vi "final.vi"() -> ()   [LabVIEW 2018]
panel:
  out "RAW\nVOLTAGE":dbl format="%#_3g"
  out "SCALED VOLTAGE":dbl(knob) scale=0.0..10.0
  in  "stop":bool
  out "STATUS":string
  out "ABOVE\nROOM\nTEMP":bool
  out "Numeric":dbl format="%#_3g"
  out "Thermometer":dbl(slide) scale=0.0..400.0
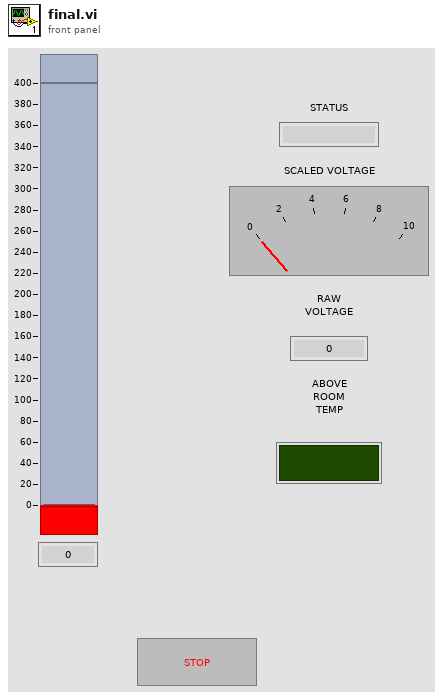
[diagram p1: front panel]
types:
  T1 = cluster{"data[0]":bool, "data[1]":bool, "data[2]":bool, "data[3]":bool, "data[4]":bool, "data[5]":bool, "data[6]":bool, "data[7]":bool, "data[8]":bool}
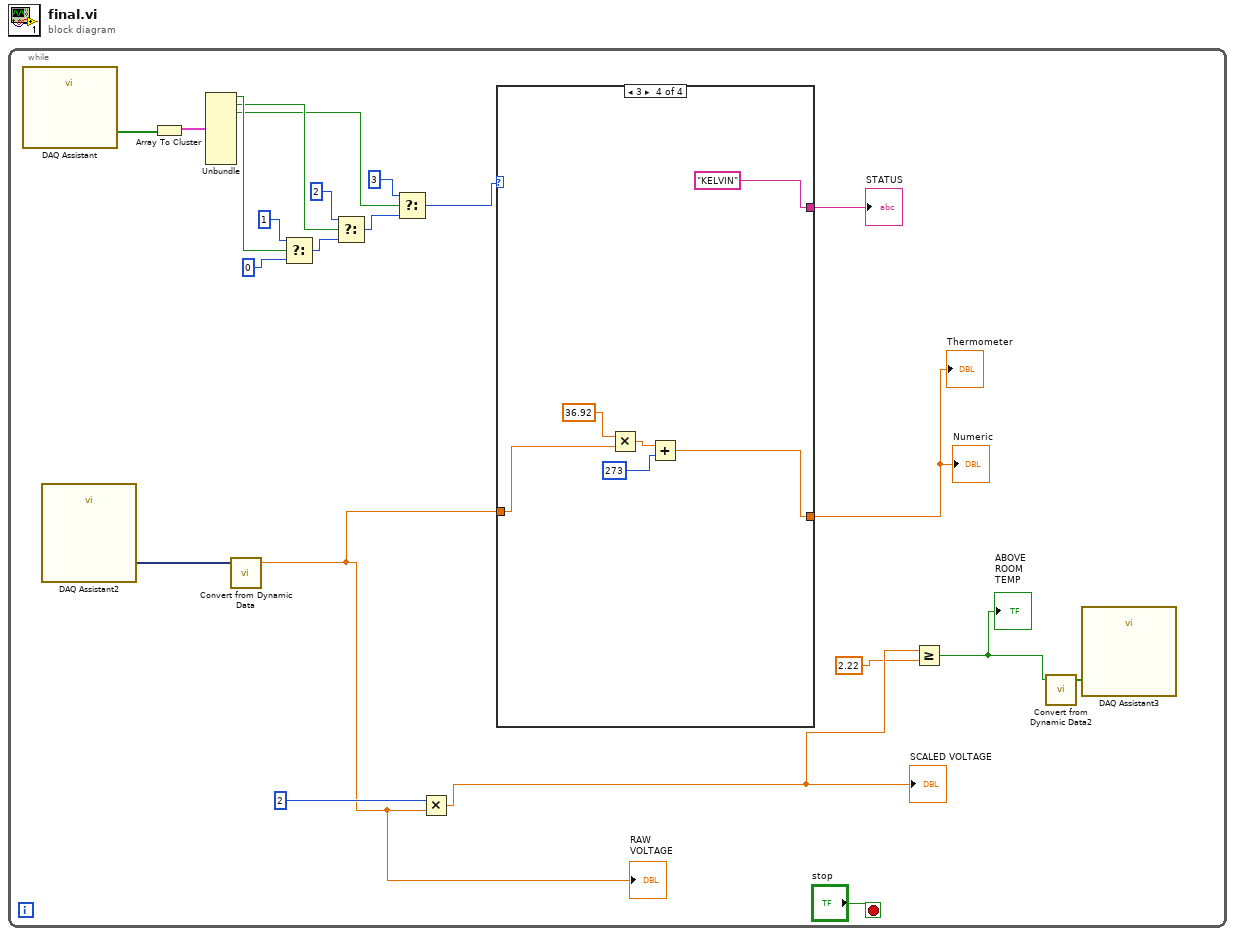
[diagram p0: block diagram]
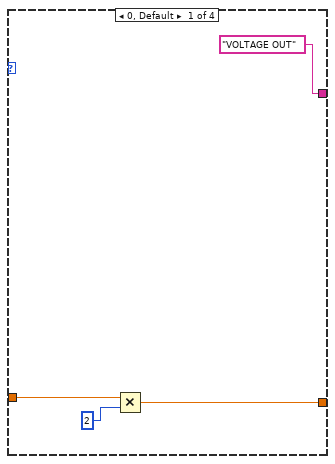
[diagram p2: hidden frame]
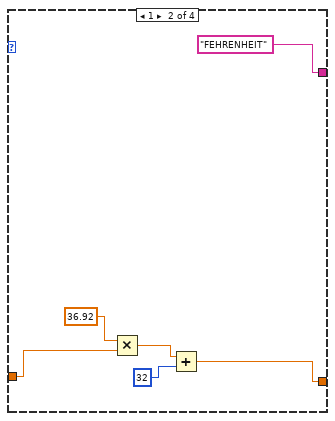
[diagram p3: hidden frame]
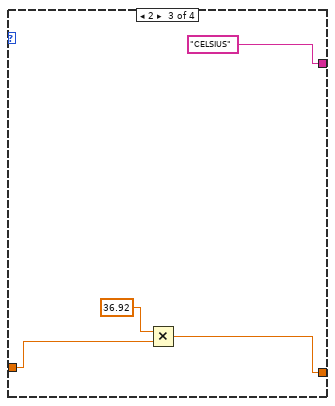
[diagram p4: hidden frame]
diagram:
  n1 = while {
    stop <- "stop" stop-if-true
    n2 = call "DAQ Assistant"() -> ("data"=w20:bool[])  [unwired: 17 in, 2 out]
    n3 = call "DAQ Assistant2"() -> ("data"=w9:dynamicdata)  [unwired: 17 in, 2 out]
    n4 = Array To Cluster(array=w20) -> (cluster=w21:T1)
    n5 = Unbundle(w21) -> ("data[0]"=w15:bool, "data[1]"=w13:bool, "data[2]"=w11:bool)  [unwired: 6 out]
    n6 = call "Convert from Dynamic Data"("Dynamic Data Type"=w9) -> ("Scalar"=w6:dbl)  [unwired: 3 in]
    "RAW\nVOLTAGE" <- w6
    n7 = Select(t=1, s=w15, f=0) -> (s? t:f=w17:i32)
    n8 = Select(t=2, s=w13, f=w17) -> (s? t:f=w16:i32)
    n9 = Select(t=3, s=w11, f=w16) -> (s? t:f=w10:i32)
    n10 = Multiply(x=2, y=w6) -> (x*y=w4:dbl)
    "SCALED VOLTAGE" <- w4
    n11 = case shown="3" w10 {
      tunnel: ["VOLTAGE OUT" "FEHRENHEIT" "CELSIUS" "KELVIN"] -> w8
      tunnel: w6 -> [w24 w31 w34 w40]
      tunnel: [w23 w27 w33 w37] -> w5
      frame 0, Default {
        n12 = Multiply(x=w24, y=2) -> (x*y=w23:dbl)
      }
      frame 1 {
        n13 = Multiply(x=36.92, y=w31) -> (x*y=w29:dbl)
        n14 = Add(x=w29, y=32) -> (x+y=w27:dbl)
      }
      frame 2 {
        n15 = Multiply(x=36.92, y=w34) -> (x*y=w33:dbl)
      }
      frame 3 {
        n16 = Multiply(x=36.92, y=w40) -> (x*y=w39:dbl)
        n17 = Add(x=w39, y=273) -> (x+y=w37:dbl)
      }
    }
    "Thermometer" <- w5
    "Numeric" <- w5
    "STATUS" <- w8
    n18 = Greater Or Equal?(x=w4, y=2.22) -> (x >= y?=w1:bool)
    "ABOVE\nROOM\nTEMP" <- w1
    n19 = call "Convert from Dynamic Data2"("Dynamic Data Type"=w1) -> ("Array"=w2:bool[])  [unwired: 3 in]
    n20 = call "DAQ Assistant3"("data"=w2) -> ()  [unwired: 17 in, 2 out]
  }
